vi "Initialize Map.vi"(10 "Column":i32, 11 "Row":i32) -> (3 "Map DVR":T1)   [LabVIEW 2015, in "Common.lvlib"]
uses:
  Common.lvlib
  Map DVR.ctl
  Location Data.ctl
  SubVIs/Read-Only Globals.vi
  SubVIs/Globals (private).vi
  Square/Square.lvclass
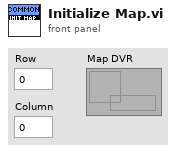
[diagram p1: front panel]
types:
  T1 = typedef "Common.lvlib/Map DVR.ctl" = refnum<data-value>
  T2 = typedef "Common.lvlib/Location Data.ctl" = cluster{"Location State":enum16{"Empty", "Enemy", "Attacked", "Occupied"}, "Round Updated":i32}
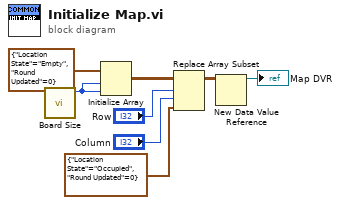
[diagram p0: block diagram]
diagram:
  n1 = call "Board Size.vi"() -> ("Board Size"=w8:i32)  [unwired: 11 in]
  n2 = Initialize Array(T2 {"Location State"=enum."Empty", "Round Updated"=0}, w8, w8) -> (w7:T2[][])
  n3 = Replace Array Subset(array=w7, new element=T2 {"Location State"=enum."Occupied", "Round Updated"=0} ("new element/subarray"), index (row)="Row", index (col)="Column") -> (w6:T2[][])
  n4 = New Data Value Reference(data value=w6) -> (data value reference=→"Map DVR":refnum<data-value>)  [unwired: 1 in, 1 out]
